vi "String to Flow device cluster.vi"(11 "FLW Device Details":string="STAT:40000000:NICK:MB0.H1:PMAX:0.1000:MAN:HVER:1:FVER:1.10:SERL:112123156:TYPE:unknown:VLIM:1:RES:10:SIG:VOLT:-0.0980V:CURR:-0.0000A:PERC:0.9613%:POWR:0.0000W") -> (3 "Flow Device Settings":T1)   [LabVIEW 2014, in "Mercury iXX.lvlib" / "Flow.lvlib"]
uses:
  Flow.lvlib
  Program Files (x86)/National Instruments/LabVIEW 2014/Public/Libraries/Flow/Controls/Flow Device (Read).ctl
  Controls/Manufacturing Data.ctl
  Controls/Flow Signals Cluster.ctl
  Mercury iXX.lvlib
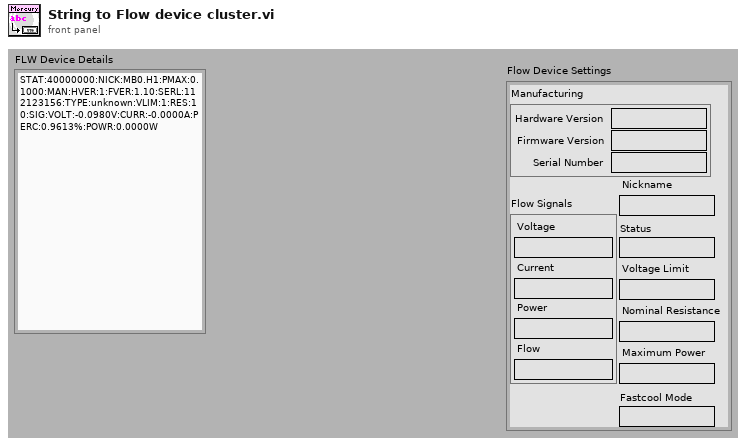
[diagram p1: front panel]
types:
  T1 = typedef "Mercury iXX.lvlib/Flow.lvlib/Flow Device (Read).ctl" = cluster{"Manufacturing":T2, "Nickname":string, "Voltage Limit":string, "Nominal Resistance":string, "Maximum Power":string, "Flow Signals":T3, "Status":string, "Fastcool Mode":string}
  T2 = typedef "Mercury iXX.lvlib/Manufacturing Data.ctl" = cluster{"Hardware Version":string, "Firmware Version":string, "Serial Number":string}
  T3 = typedef "Mercury iXX.lvlib/Flow.lvlib/Flow Signals Cluster.ctl" = cluster{"Voltage":string, "Current":string, "Power":string, "Flow":string}
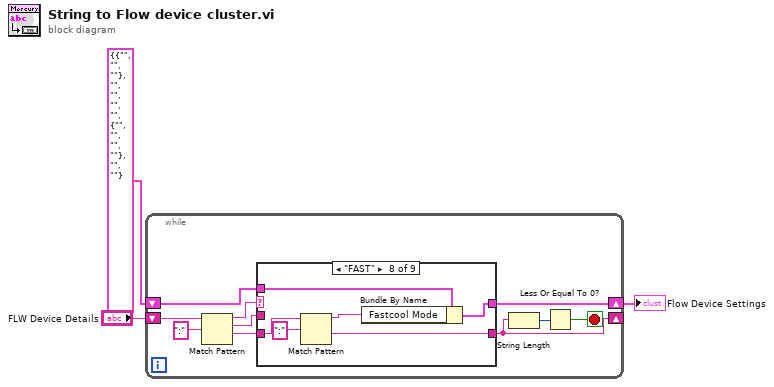
[diagram p0: block diagram]
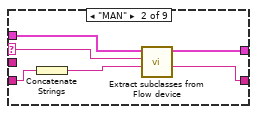
[diagram p3: hidden frame]
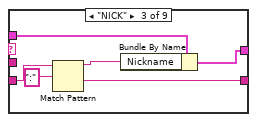
[diagram p4: hidden frame]
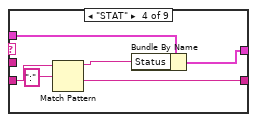
[diagram p5: hidden frame]
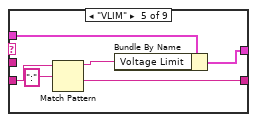
[diagram p6: hidden frame]
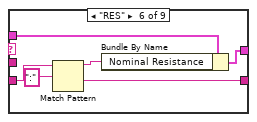
[diagram p7: hidden frame]
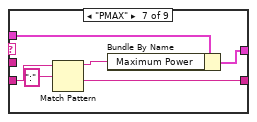
[diagram p8: hidden frame]
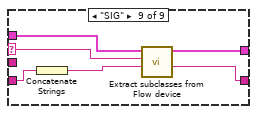
[diagram p9: hidden frame]
diagram:
  n1 = while {
    shift-right: [w9] -> w2
    shift-left: T1 {"Manufacturing"={"Hardware Version"="", "Firmware Version"="", "Serial Number"=""}, "Nickname"="", "Voltage Limit"="", "Nominal Resistance"="", "Maximum Power"="", "Flow Signals"={"Voltage"="", "Current"="", "Power"="", "Flow"=""}, "Status"="", "Fastcool Mode"=""} ("Heater Device Settings") -> [w10]
    shift-right: [w5] -> _
    shift-left: "FLW Device Details" -> [w12]
    stop <- w4 stop-if-true
    n2 = Match Pattern(string=w12, regular expression=":") -> (before substring=w11:string, match substring=w8:string, after substring=w7:string)  [unwired: 2 out]
    n3 = case shown="\"FAST\"" w11 {
      selector: w11 -> [_ w21 _ _ _ _ _ _ w63]
      tunnel: w8 -> [_ _ _ _ _ _ _ _ _]
      tunnel: w10 -> [w15 w17 w25 w31 w37 w43 w49 w55 w59]
      tunnel: [w15 w16 w24 w30 w36 w42 w48 w54 w58] -> w9
      tunnel: [w14 w20 w22 w28 w34 w40 w46 w52 w62] -> w5
      tunnel: w7 -> [w14 w18 w26 w32 w38 w44 w50 w56 w60]
      frame "", Default {
      }
      frame "MAN" {
        n4 = Concatenate Strings(w18) -> (w19:string)
        n5 = call "Extract subclasses from Flow device.vi"("Data In"=w19, "Class"=w21, "Heater Device Settings in"=w17) -> ("Data out"=w20:string, "Heater Device Settings out"=w16:T1)  [unwired: 1 in, 6 out]
      }
      frame "NICK" {
        n6 = Match Pattern(string=w26, regular expression=":") -> (before substring=w23:string, after substring=w22:string)  [unwired: 3 out]
        n7 = Bundle By Name(cluster=w25, "Nickname"=w23) -> (w24:T1)
      }
      frame "STAT" {
        n8 = Match Pattern(string=w32, regular expression=":") -> (before substring=w29:string, after substring=w28:string)  [unwired: 3 out]
        n9 = Bundle By Name(cluster=w31, "Status"=w29) -> (w30:T1)
      }
      frame "VLIM" {
        n10 = Match Pattern(string=w38, regular expression=":") -> (before substring=w35:string, after substring=w34:string)  [unwired: 3 out]
        n11 = Bundle By Name(cluster=w37, "Voltage Limit"=w35) -> (w36:T1)
      }
      frame "RES" {
        n12 = Match Pattern(string=w44, regular expression=":") -> (before substring=w41:string, after substring=w40:string)  [unwired: 3 out]
        n13 = Bundle By Name(cluster=w43, "Nominal Resistance"=w41) -> (w42:T1)
      }
      frame "PMAX" {
        n14 = Match Pattern(string=w50, regular expression=":") -> (before substring=w47:string, after substring=w46:string)  [unwired: 3 out]
        n15 = Bundle By Name(cluster=w49, "Maximum Power"=w47) -> (w48:T1)
      }
      frame "FAST" {
        n16 = Match Pattern(string=w56, regular expression=":") -> (before substring=w53:string, after substring=w52:string)  [unwired: 3 out]
        n17 = Bundle By Name(cluster=w55, "Fastcool Mode"=w53) -> (w54:T1)
      }
      frame "SIG" {
        n18 = Concatenate Strings(w60) -> (w61:string)
        n19 = call "Extract subclasses from Flow device.vi"("Data In"=w61, "Class"=w63, "Heater Device Settings in"=w59) -> ("Data out"=w62:string, "Heater Device Settings out"=w58:T1)  [unwired: 1 in, 6 out]
      }
    }
    n20 = String Length(string=w5) -> (length=w6:i32)
    n21 = Less Or Equal To 0?(x=w6) -> (x <= 0?=w4:bool)
  }
  "Flow Device Settings" <- w2
